vi "checkFinishBallOutOfFieldPlay.vi"(8 "error in (no error)":errorcluster, 10 "Game":refnum<class "Game.lvclass">, 11 "BallOutOfFieldPlay in":refnum<class "BallOutOfFieldPlay.lvclass">) -> (0 "error out":errorcluster, 2 "Finish Ball Out?":bool, 3 "BallOutOfFieldPlay out":refnum<class "BallOutOfFieldPlay.lvclass">)   [LabVIEW 2023, in "BallOutOfFieldPlay.lvclass"]
uses:
  BallOutOfFieldPlay.lvclass
  Game_class/Game.lvclass
  Game_class/Game.lvclass/Game.ctl
  Events_class/Events.lvclass/Events.ctl
  Game_class/Read EventsRef.vi
  Events_class/Read ball_out.vi
  Events_class/Events.lvclass
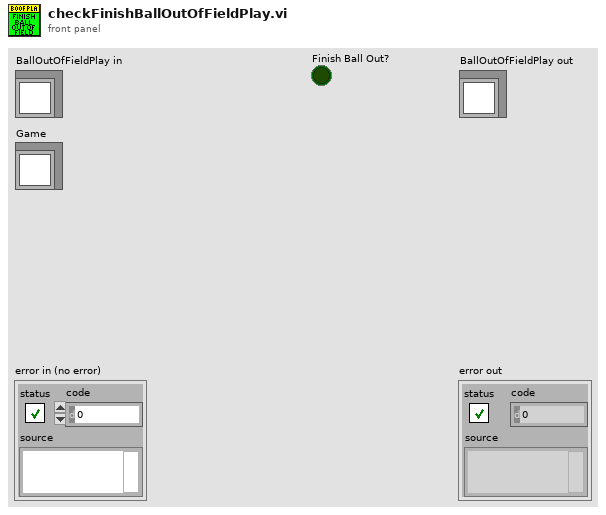
[diagram p1: front panel]
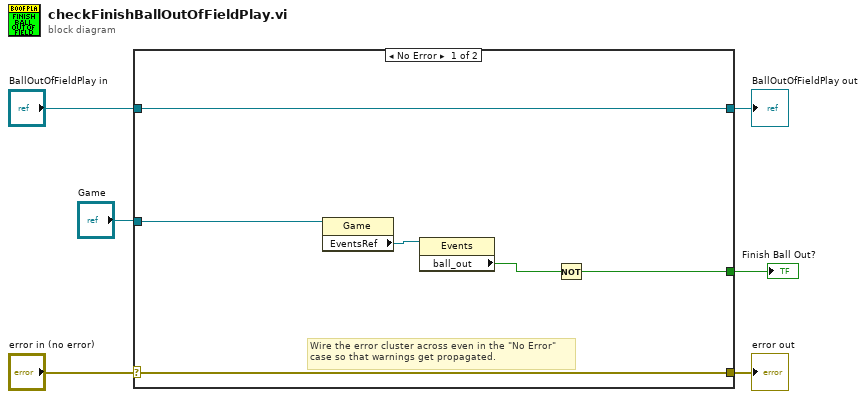
[diagram p0: block diagram]
diagram:
  n1 = case shown="No Error" "error in (no error)" {
    selector: "error in (no error)" -> [w11 w14]
    tunnel: [w11 w14] -> w5
    tunnel: [w12 w13] -> w3
    tunnel: "BallOutOfFieldPlay in" -> [w12 w13]
    tunnel: "Game" -> [w10 _]
    tunnel: [w7 _] -> w1
    frame No Error {
      # "Wire the error cluster across even in the \"No Error\"\ncase so that warnings get propagated."
      n2 = property class="Game"(reference=w10) -> ("EventsRef"=w9:refnum<class "Events.lvclass">)  [unwired: 1 in, 2 out]
      n3 = property class="Events"(reference=w9) -> ("ball_out"=w8:bool)  [unwired: 1 in, 2 out]
      n4 = Not(x=w8) -> (.not. x?=w7:bool)
    }
    frame Error {
    }
  }
  "error out" <- w5
  "BallOutOfFieldPlay out" <- w3
  "Finish Ball Out?" <- w1
